vi "Project V50 Report (SubVI).vi"(8 "errIN":errorcluster, 9 "pastPanels":string[][](array[string]), 10 "prjSelect":bool[](array[boolean]), 11 "Project ID":refnum<vi>) -> (0 "errOUT":errorcluster)   [LabVIEW 2015]
uses:
  <vilib>/Utility/NIReport.llb/NI_report.lvclass
  <vilib>/Utility/NIReport.llb/Excel/NI_Excel.lvclass
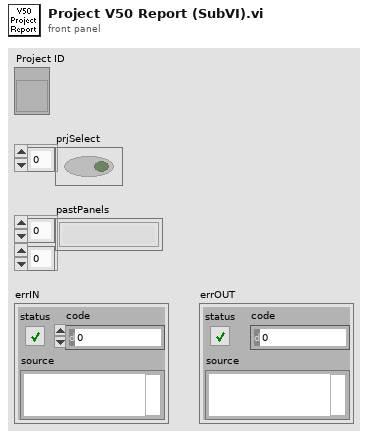
[diagram p1: front panel]
types:
  T1 = enum16{"maximized", "minimized", "normal", "no change"}
  T2 = enum16{"Standard Report", "HTML", "Word", "Excel"}
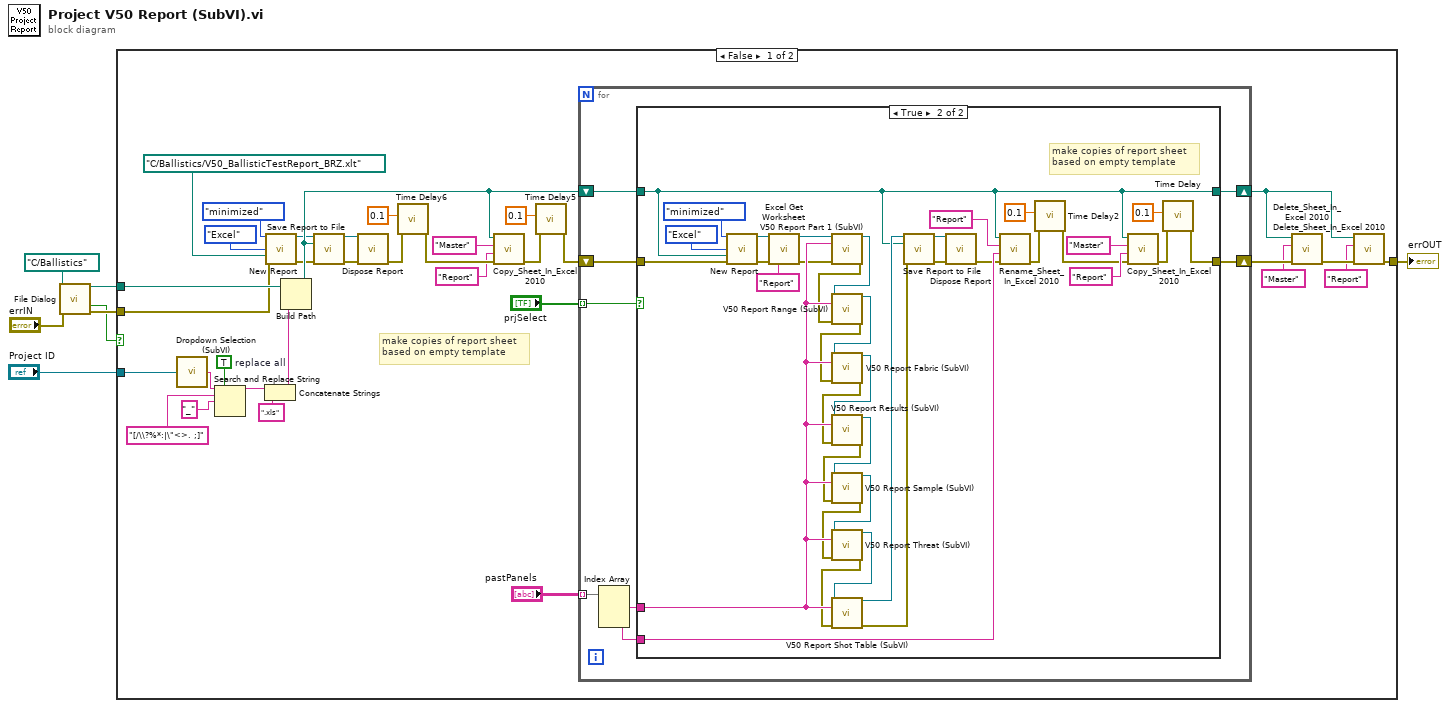
[diagram p0: block diagram]
diagram:
  n1 = call "File Dialog"("start path"=path "C:/Ballistics" ("Custom Template"), "error in"="errIN") -> ("selected path"=w4:path, "cancelled"=w1:bool, "error out"=w2:errorcluster)  [unwired: 10 in, 1 out]
  n2 = case shown="False" w1 {
    tunnel: "Project ID" -> [w32 _]
    tunnel: [w11 w89] -> w6
    tunnel: w4 -> [w9 _]
    tunnel: w2 -> [w8 w89]
    frame False {
      w38 = TRUE  # replace all
      # "make copies of report sheet\nbased on empty template"
      n3 = call "Dropdown Selection (SubVI).vi"("reference"=w32) -> ("element"=w36:string)
      n4 = Search and Replace String(replace all?=w38, input string=w36, search string="[/\\?%*:|\"<>. ;]", replace string="_" ("replace string (\"\")")) -> (result string=w39:string)  [unwired: 4 in, 3 out]
      n5 = Concatenate Strings(w39, ".xls" ("string")) -> (w33:string)
      n6 = call <vilib>:"New Report.vi"("window state (normal)"=T1."minimized", "report type"=T2."Excel", "template (empty)"=path "C:/Ballistics/V50_BallisticTestReport_BRZ.xlt" ("Custom Template"), "error in (no error)"=w8) -> ("report out"=w17:refnum<class "NI_report.lvclass">, "error out"=w16:errorcluster)  [unwired: 10 in]
      n7 = Build Path(base path=w9, name or relative path=w33) -> (appended path=w18:path)
      n8 = call-dynamic "Save Report to File.vi"("report in"=w17, "report file path"=w18, "error in (no error)"=w16) -> ("report out"=w27:refnum<class "NI_report.lvclass">, "error out"=w28:errorcluster)  [unwired: 11 in]
      n9 = call-dynamic "Dispose Report.vi"("report in"=w27, "error in (no error)"=w28) -> ("error out"=w29:errorcluster)  [unwired: 13 in]
      n10 = call "Time Delay6"("error in (no error)"=w29, "Delay Time (s)"=0.1) -> ("error out"=w23:errorcluster)  [unwired: 9 in]
      n11 = call "Copy_Sheet_In_Excel 2010.vi"("error in (no error)"=w23, "New Sheet Name"="Report", "Master Sheet Name"="Master" ("New Sheet Name"), "Excel Path"=w18) -> ("error out"=w26:errorcluster)  [unwired: 7 in]
      n12 = call "Time Delay5"("error in (no error)"=w26, "Delay Time (s)"=0.1) -> ("error out"=w19:errorcluster)  [unwired: 9 in]
      n13 = for {
        tunnel: "prjSelect" -> [w49] mode=indexing
        tunnel: "pastPanels" -> [w46] mode=indexing
        shift-right: [w48] -> w41
        shift-left: w19 -> [w43]
        shift-right: [w47] -> w13
        shift-left: w18 -> [w42]
        n14 = Index Array(array=w46) -> (element #1=w45:string, element #3=w44:string)  [unwired: 3 in, 1 out]
        n15 = case shown="True" w49 {
          tunnel: w43 -> [w51 w85]
          tunnel: [w51 w65] -> w48
          tunnel: w42 -> [w50 w64]
          tunnel: [w50 w64] -> w47
          tunnel: w45 -> [_ w80]
          tunnel: w44 -> [_ w76]
          frame False {
          }
          frame True {
            # "make copies of report sheet\nbased on empty template"
            n16 = call <vilib>:"New Report.vi"("window state (normal)"=T1."minimized", "report type"=T2."Excel", "template (empty)"=w64, "error in (no error)"=w85) -> ("report out"=w84:refnum<class "NI_report.lvclass">, "error out"=w83:errorcluster)  [unwired: 10 in]
            n17 = call <vilib>:"Excel Get Worksheet.vi"("report in"=w84, "error in (no error)"=w83, "name (\"\")"="Report" ("New Sheet Name")) -> ("report out"=w78:refnum<class "NI_report.lvclass">, "error out"=w79:errorcluster)  [unwired: 11 in]
            n18 = call "V50 Report Part 1 (SubVI).vi"("NI_report in"=w78, "SampleID"=w80, "error in (no error)"=w79) -> ("NI_report out"=w62:refnum<class "NI_report.lvclass">, "error out"=w63:errorcluster)  [unwired: 11 in]
            n19 = call "V50 Report Range (SubVI).vi"("NI_report in"=w62, "SampleID"=w80, "error in (no error)"=w63) -> ("NI_report out"=w60:refnum<class "NI_report.lvclass">, "error out"=w61:errorcluster)  [unwired: 11 in]
            n20 = call "V50 Report Fabric (SubVI).vi"("NI_report in"=w60, "SampleID"=w80, "error in (no error)"=w61) -> ("NI_report out"=w58:refnum<class "NI_report.lvclass">, "error out"=w59:errorcluster)  [unwired: 11 in]
            n21 = call "V50 Report Results (SubVI).vi"("NI_report in"=w58, "SampleID"=w80, "error in (no error)"=w59) -> ("NI_report out"=w56:refnum<class "NI_report.lvclass">, "error out"=w57:errorcluster)  [unwired: 11 in]
            n22 = call "V50 Report Sample (SubVI).vi"("NI_report in"=w56, "SampleID"=w80, "error in (no error)"=w57) -> ("NI_report out"=w54:refnum<class "NI_report.lvclass">, "error out"=w55:errorcluster)  [unwired: 11 in]
            n23 = call "V50 Report Threat (SubVI).vi"("NI_report in"=w54, "SampleID"=w80, "error in (no error)"=w55) -> ("NI_report out"=w52:refnum<class "NI_report.lvclass">, "error out"=w53:errorcluster)  [unwired: 11 in]
            n24 = call "V50 Report Shot Table (SubVI).vi"("NI_report in"=w52, "SampleID"=w80, "error in (no error)"=w53) -> ("NI_report out"=w74:refnum<class "NI_report.lvclass">, "error out"=w73:errorcluster)  [unwired: 11 in]
            n25 = call-dynamic "Save Report to File.vi"("report in"=w74, "report file path"=w64, "error in (no error)"=w73) -> ("report out"=w87:refnum<class "NI_report.lvclass">, "error out"=w86:errorcluster)  [unwired: 11 in]
            n26 = call-dynamic "Dispose Report.vi"("report in"=w87, "error in (no error)"=w86) -> ("error out"=w75:errorcluster)  [unwired: 13 in]
            n27 = call "Rename_Sheet_In_Excel 2010.vi"("error in (no error)"=w75, "New Sheet Name"=w76, "Master Sheet Name"="Report" ("New Sheet Name"), "Excel Path"=w64) -> ("error out"=w66:errorcluster)  [unwired: 7 in]
            n28 = call "Time Delay2"("error in (no error)"=w66, "Delay Time (s)"=0.1) -> ("error out"=w70:errorcluster)  [unwired: 9 in]
            n29 = call "Copy_Sheet_In_Excel 2010.vi"("error in (no error)"=w70, "New Sheet Name"="Report", "Master Sheet Name"="Master" ("New Sheet Name"), "Excel Path"=w64) -> ("error out"=w67:errorcluster)  [unwired: 7 in]
            n30 = call "Time Delay"("error in (no error)"=w67, "Delay Time (s)"=0.1) -> ("error out"=w65:errorcluster)  [unwired: 9 in]
          }
        }
      }
      n31 = call "Delete_Sheet_In_Excel 2010.vi"("error in (no error)"=w41, "Master Sheet Name"="Master" ("New Sheet Name"), "Excel Path"=w13) -> ("error out"=w12:errorcluster)  [unwired: 8 in]
      n32 = call "Delete_Sheet_In_Excel 2010.vi"("error in (no error)"=w12, "Master Sheet Name"="Report" ("New Sheet Name"), "Excel Path"=w13) -> ("error out"=w11:errorcluster)  [unwired: 8 in]
    }
    frame True {
      # "canceled"
    }
  }
  "errOUT" <- w6
